vi "Write Conversion Time.vi"(8 "error in":errorcluster, 10 "conversion time":T1, 11 "NI 9213 in":refnum<class "NI 9213.lvclass">) -> (0 "error out":errorcluster, 3 "NI 9213 out":refnum<class "NI 9213.lvclass">)   [LabVIEW 2017, in "Scan Engine Scripting.lvlib" / "NI 9213.lvclass"]
doc: "Writes the conversion time to the module private data."
uses:
  NI 9213.lvclass
  NI 9213 Conversion Time.ctl
  NI 9213.lvclass/NI 9213.ctl
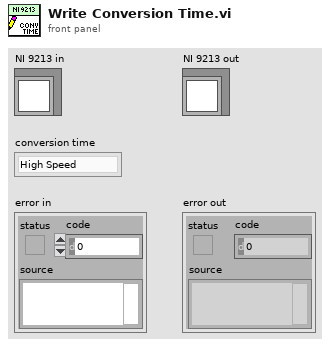
[diagram p1: front panel]
types:
  T1 = typedef "Scan Engine Scripting.lvlib/NI 9213.lvclass/NI 9213 Conversion Time.ctl" = enum16{"High Speed", "High Resolution"}
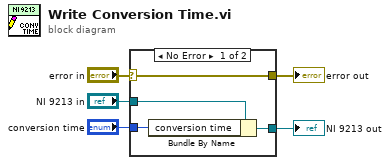
[diagram p0: block diagram]
diagram:
  n1 = case shown="No Error" "error in" {
    selector: "error in" -> [w9 w10]
    tunnel: [w9 w10] -> w4
    tunnel: [w7 w11] -> w1
    tunnel: "NI 9213 in" -> [w8 w11]
    tunnel: "conversion time" -> [w6 _]
    frame No Error {
      n2 = Bundle By Name(cluster=w8, "conversion time"=w6) -> (w7:refnum<class "NI 9213.lvclass">)
    }
    frame Error {
    }
  }
  "error out" <- w4
  "NI 9213 out" <- w1
